vi "Prueba_runastartup.vi"() -> ()   [LabVIEW 2015]
uses:
  <vilib>/NI_Real-Time Target Support.lvlib
panel:
  in  "stop":bool
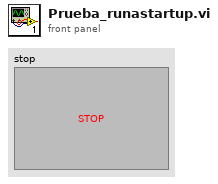
[diagram p1: front panel]
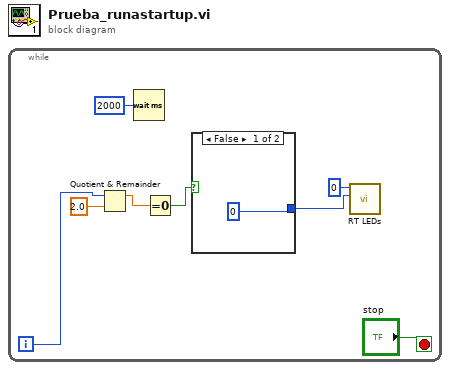
[diagram p0: block diagram]
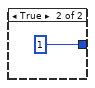
[diagram p2: hidden frame]
diagram:
  n1 = while {
    i -> [w5]
    stop <- "stop" stop-if-true
    n2 = Quotient & Remainder(x=w5, y=2.0) -> (x-y*floor(x/y)=w1:dbl)  [unwired: 1 out]
    n3 = Wait (ms)(milliseconds to wait=u32 2000) -> ()  [unwired: 1 out]
    n4 = Equal To 0?(x=w1) -> (x = 0?=w4:bool)
    n5 = case shown="False" w4 {
      tunnel: [0 ("LED Num") 1 ("State")] -> w3
      frame False {
      }
      frame True {
      }
    }
    n6 = call <vilib>:"RT LEDs.vi"("State"=w3, "LED Num"=0) -> ()  [unwired: 1 in, 5 out]
  }
